vi "PathPlanner_EventMarker_ShouldTrigger.vi"(9 "RobotPose":T5={"TRANSLATION"={"X"=0.0, "Y"=0.0}, "ROTATION"={"VALUE"=0.0, "COS"=1.0, "SIN"=0.0}} {"ROTATION"."SIN" format="%13.4f"; "ROTATION"."COS" format="%13.4f"; "ROTATION"."VALUE" format="%13.4f"; "TRANSLATION"."Y" format="%14.3f"; "TRANSLATION"."X" format="%14.3f"}, 11 "in EventMarker":T1 {"lastRobotPos"."Y" format="%14.3f"; "lastRobotPos"."X" format="%14.3f"; "markerPos"."Y" format="%14.3f"; "markerPos"."X" format="%14.3f"}) -> (1 "ShouldTrigger":bool, 3 "out EventMarker":T1 {"lastRobotPos"."Y" format="%14.3f"; "lastRobotPos"."X" format="%14.3f"; "markerPos"."Y" format="%14.3f"; "markerPos"."X" format="%14.3f"})   [LabVIEW 2019, in "PathPlanner.lvlib"]
doc: "Get if this event marker should be triggered\n\nInputs:\n - EventMarker - cluster - Data cluster\n - robotPose - pose2d - Current pose of the robot\n\nOutputs:\n - EventMarker - cluster - Data cluster\n - Trigger - boolean - True if this marker should be triggered"
uses:
  PathPlanner.lvlib
  TypeDef/PathPlannerEventMarker.ctl
  <vilib>/Rock Robotics/WPI/ThirdParty/JAS_Junk/TrajLib/TypeDef/TRANSLATION2D.ctl
  TypeDef/PathPlannerCommandUtil.ctl
  ENum/PathPlanner_CommandUtilType_ENUM.ctl
  <vilib>/Rock Robotics/WPI/ThirdParty/JAS_Junk/TrajLib/TypeDef/POSE2D.ctl
  <vilib>/Rock Robotics/WPI/ThirdParty/JAS_Junk/TrajLib/TypeDef/ROTATION2D.ctl
  <vilib>/Rock Robotics/WPI/ThirdParty/JAS_Junk/TrajLib/Util_CalcDist.vi
  <vilib>/Rock Robotics/WPI/ThirdParty/JAS_Junk/TrajLib/Trajectory_Library.lvlib
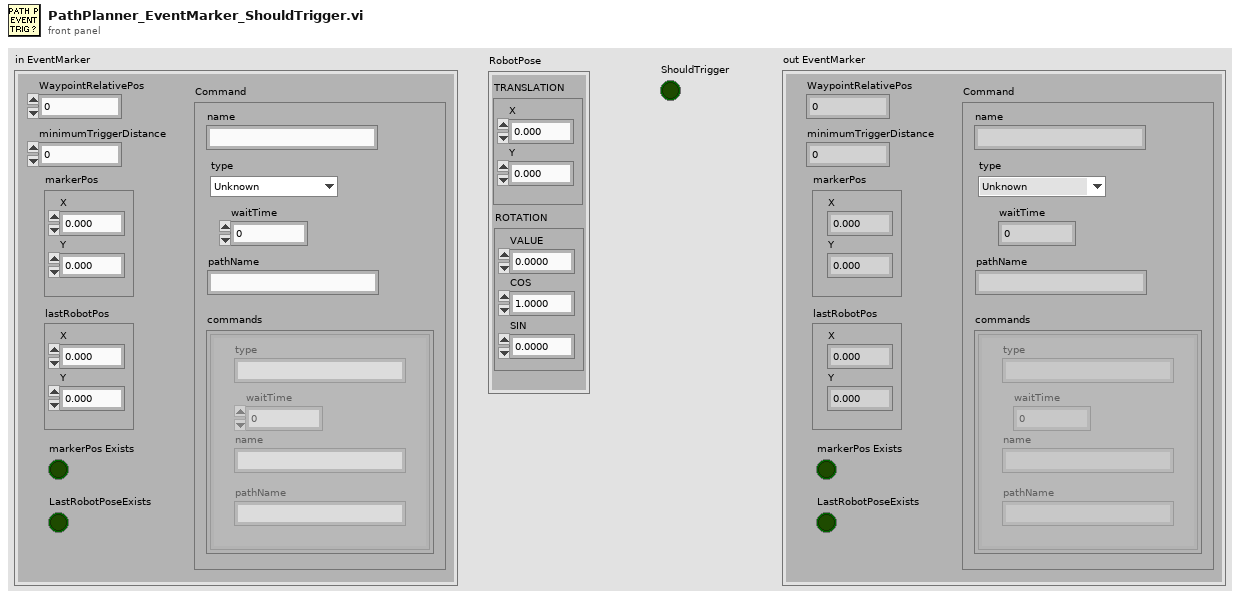
[diagram p1: front panel]
types:
  T1 = typedef "PathPlanner.lvlib/PathPlannerEventMarker.ctl" = cluster{"WaypointRelativePos":dbl, "minimumTriggerDistance":dbl, "markerPos":T2, "lastRobotPos":T2, "Command":T3, "markerPos Exists":bool, "LastRobotPoseExists":bool}
  T2 = typedef "Trajectory_Library.lvlib/TRANSLATION2D.ctl" = cluster{"X":dbl, "Y":dbl}
  T3 = typedef "PathPlanner.lvlib/PathPlannerCommandUtil.ctl" = cluster{"waitTime":dbl, "name":string, "pathName":string, "commands":cluster{"type":string, "waitTime":dbl, "name":string, "pathName":string}[], "type":T4}
  T4 = typedef "PathPlanner.lvlib/PathPlanner_CommandUtilType_ENUM.ctl" = enum16{"Unknown", "Wait", "Named", "Path", "Sequential", "Parallel", "Race", "Deadline"}
  T5 = typedef "Trajectory_Library.lvlib/POSE2D.ctl" = cluster{"TRANSLATION":T2, "ROTATION":T6}
  T6 = typedef "Trajectory_Library.lvlib/ROTATION2D.ctl" = cluster{"VALUE":dbl, "COS":dbl, "SIN":dbl}
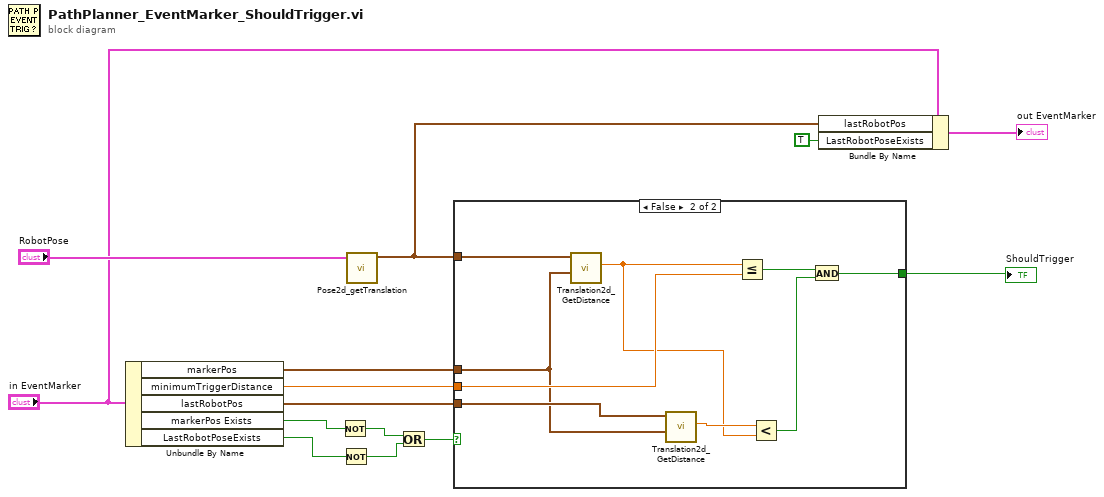
[diagram p0: block diagram]
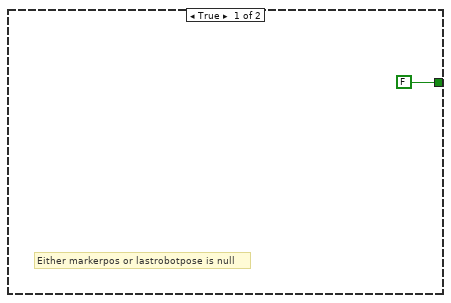
[diagram p2: hidden frame]
diagram:
  n1 = Unbundle By Name("in EventMarker") -> ("markerPos"=w12:T2, "minimumTriggerDistance"=w14:dbl, "lastRobotPos"=w13:T2, "markerPos Exists"=w10:bool, "LastRobotPoseExists"=w9:bool)
  n2 = Not(x=w10) -> (.not. x?=w8:bool)
  n3 = Not(x=w9) -> (.not. x?=w7:bool)
  n4 = call <vilib>:"Pose2d_getTranslation.vi"("in POSE"="RobotPose") -> ("outTRANSLATION"=w5:T2)  [unwired: 10 in]
  n5 = Or(x=w8, y=w7) -> (x .or. y?=w2:bool)
  n6 = case shown="False" w2 {
    tunnel: w14 -> [_ w24]
    tunnel: w13 -> [_ w22]
    tunnel: w12 -> [_ w21]
    tunnel: [FALSE w17] -> w11
    tunnel: w5 -> [_ w16]
    frame True {
      # "Either markerpos or lastrobotpose is null"
    }
    frame False {
      n7 = call <vilib>:"Translation2d_GetDistance.vi"("other Translation"=w21, "In Translation"=w16) -> ("Distance"=w19:dbl)  [unwired: 9 in]
      n8 = call <vilib>:"Translation2d_GetDistance.vi"("other Translation"=w21, "In Translation"=w22) -> ("Distance"=w20:dbl)  [unwired: 9 in]
      n9 = Less Or Equal?(x=w19, y=w24) -> (x <= y?=w23:bool)
      n10 = Less?(x=w20, y=w19) -> (x < y?=w18:bool)
      n11 = And(x=w23, y=w18) -> (x .and. y?=w17:bool)
    }
  }
  "ShouldTrigger" <- w11
  n12 = Bundle By Name(cluster="in EventMarker", "lastRobotPos"=w5, "LastRobotPoseExists"=TRUE) -> (→"out EventMarker":T1)
